vi "Get-motor-by-index.vi"(8 "error in (no error)":errorcluster, 10 "Index":i32, 11 "Available motors in":refnum<class "Motor-assembly.lvclass">) -> (0 "error out":errorcluster, 1 "Active?":bool, 2 "Motor":refnum<class "Motor.lvclass">, 3 "Available motors out":refnum<class "Motor-assembly.lvclass">)   [LabVIEW 2013, in "PowderDeposition.lvlib" / "Motor-assembly.lvclass"]
uses:
  Motor-assembly.lvclass
  Motor/Motor.lvclass
  Motor-assembly.lvclass/Motor-assembly.ctl
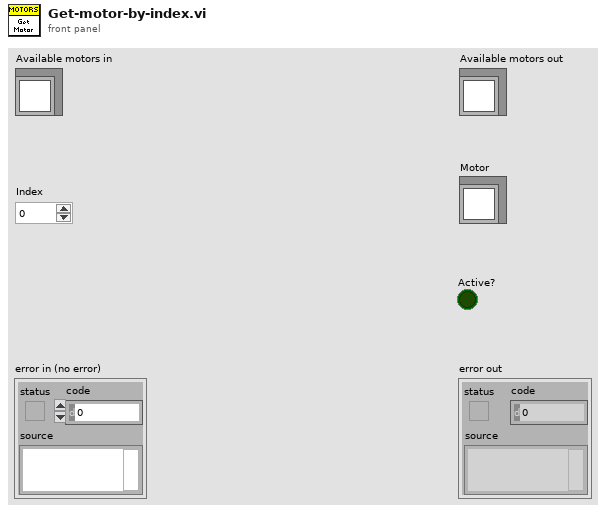
[diagram p1: front panel]
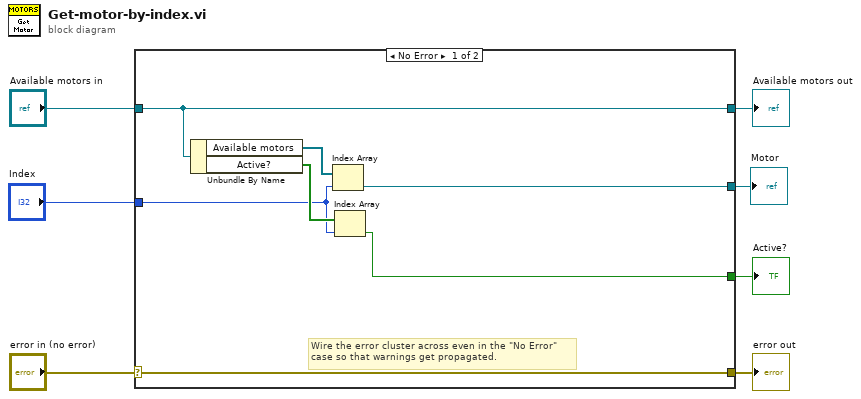
[diagram p0: block diagram]
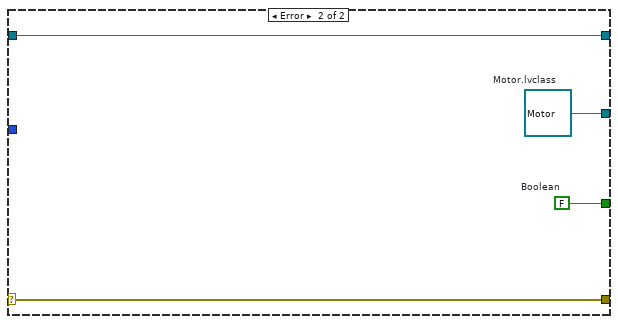
[diagram p2: hidden frame]
diagram:
  n1 = case shown="No Error" "error in (no error)" {
    selector: "error in (no error)" -> [w14 w18]
    tunnel: [w14 w18] -> w6
    tunnel: [w13 w17] -> w4
    tunnel: "Available motors in" -> [w13 w17]
    tunnel: "Index" -> [w9 _]
    tunnel: [w11 w16] -> w2
    tunnel: [w8 w15] -> w1
    frame No Error {
      # "Wire the error cluster across even in the \"No Error\"\ncase so that warnings get propagated."
      n2 = Unbundle By Name(w13) -> ("Available motors"=w12:refnum<class "Motor.lvclass">[], "Active?"=w10:bool[])
      n3 = Index Array(array=w12, index=w9) -> (element=w11:refnum<class "Motor.lvclass">)
      n4 = Index Array(array=w10, index=w9) -> (element=w8:bool)
    }
    frame Error {
      w15 = FALSE  # Boolean
      w16 = refnum<class "Motor.lvclass"> refnum  # Motor.lvclass
    }
  }
  "error out" <- w6
  "Available motors out" <- w4
  "Motor" <- w2
  "Active?" <- w1
